vi "Teleop.vi"(10 "Match Info":T1={"Autonomous Elapsed Seconds"=0.0, "TeleOp Elapsed Seconds"=0.0, "Disabled Elapsed Seconds"=0.0, "Visited Autonomous"=FALSE, "Visited TeleOp"=FALSE, "Visited Disabled"=FALSE, "Autonomous Settings"={"Autonomous Style"=enum."Independent", "VI Refnum"=refnum}}, 11 "Call Context":T2) -> ()   [LabVIEW 2015]
doc: "This VI is called for each TeleOp packet received from the DS where the robot is not disabled. It is often used to read from the joysticks and update I/O or to update setpoints for timed control loops. It should complete and return within 20 milliseconds or it may miss DS packets."
uses:
  <vilib>/Rock Robotics/WPI/DriverStation/WPI_DriverStationDerivedRobotMode.ctl
  <vilib>/Rock Robotics/WPI/DriverStation/WPI_DriverStationMatch Info.ctl
  <vilib>/Rock Robotics/WPI/Solenoid/WPI_SolenoidValue.ctl
  <vilib>/Rock Robotics/WPI/Utilities/WPI_GetSetVariantRefNum.vi
  <vilib>/Rock Robotics/Network Tables/NT Write Boolean Array.vi
  <vilib>/Rock Robotics/Network Tables/NT Write Numeric Array.vi
  <vilib>/Rock Robotics/Network Tables/NT Read Boolean.vi
  <vilib>/Rock Robotics/Network Tables/NT Read Number.vi
  Robot Global Data.vi
  <vilib>/Rock Robotics/WPI/Solenoid/WPI_SolenoidSetEnum.vi
panel:
  out "Sample Slider 0":dbl(slide) scale=0.0..5.0
  out "Sample Boolean 1":bool
  out "Sample Boolean 0":bool
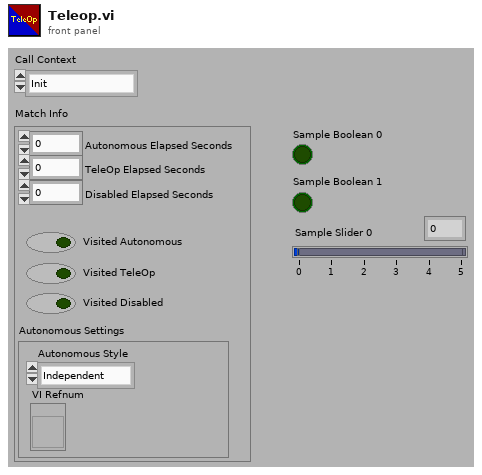
[diagram p1: front panel]
types:
  T1 = typedef "WPI_DriverStationMatch Info.ctl" = cluster{"Autonomous Elapsed Seconds":dbl, "TeleOp Elapsed Seconds":dbl, "Disabled Elapsed Seconds":dbl, "Visited Autonomous":bool, "Visited TeleOp":bool, "Visited Disabled":bool, "Autonomous Settings":cluster{"Autonomous Style":enum16{"Iterative", "Independent"}, "VI Refnum":refnum<vi>}}
  T2 = typedef "WPI_DriverStationDerivedRobotMode.ctl" = enum16{"Init", "Execute", "Stop"}
  T3 = typedef "WPI_JoystickDevRef.ctl" = cluster{"Device":T4}
  T4 = typedef "WPI_JoystickDeviceEnum.ctl" = enum16{"USB 0", "USB 1", "USB 2", "USB 3", "USB 4", "USB 5"}
  T5 = cluster{"Buttons[0]":bool, "Buttons[1]":bool, "Buttons[2]":bool, "Buttons[3]":bool, "Buttons[4]":bool, "Buttons[5]":bool, "Buttons[6]":bool, "Buttons[7]":bool, "Buttons[8]":bool}
  T6 = cluster{"Axes[0]":dbl, "Axes[1]":dbl, "Axes[2]":dbl, "Axes[3]":dbl, "Axes[4]":dbl, "Axes[5]":dbl, "Axes[6]":dbl, "Axes[7]":dbl, "Axes[8]":dbl}
  T7 = typedef "WPI_RobotDriveDevRef.ctl" = cluster{"DevStatus":errorcluster, "Motors[]":T8[], "Square Inputs":bool, "Max Output":dbl}
  T8 = typedef "WPI_MotorControlDeviceRef.ctl" = cluster{"DeviceStatus":errorcluster, "Type":T9, "PWM":cluster{"PWM Channel":T10, "DeadBand":T11}, "CAN":cluster{"Device Number":u8, "Control Mode":T12, "Semaphore":T13, "Max Vout":dbl, "TalonSRX Control Mode":T14}, "Invert":bool}
  T9 = typedef "WPI_MotorControlType.ctl" = enum16{"PWM", "CAN", "CANTalonSRX"}
  T10 = typedef "FPGA_DIOPWMChannel.ctl" = enum8{"PWM 0", "PWM 1", "PWM 2", "PWM 3", "PWM 4", "PWM 5", "PWM 6", "PWM 7", "PWM 8", "PWM 9", "PWM MXP 0", "PWM MXP 1", "PWM MXP 2", "PWM MXP 3", "PWM MXP 4", "PWM MXP 5", "PWM MXP 6", "PWM MXP 7", "PWM MXP 8", "PWM MXP 9", "Invalid"}
  T11 = typedef "WPI_PWMDeadband.ctl" = cluster{"Name":string, "maxPositivePwm":i32, "minPositivePwm":i32, "centerPwm":i32, "maxNegativePwm":i32, "minNegativePwm":i32, "angularRange":u16}
  T12 = typedef "WPI_CANJaguar_ControlMode.ctl" = enum8{"Percent VBus", "Current", "Speed", "Position", "Voltage"}
  T13 = typedef "Semaphore RefNum" = refnum<k1>
  T14 = typedef "WPI_CANTalonSRX_APIControlMode.ctl" = enum8{"Percent VBus", "Speed", "Position", "Slave", "Unchanged / Invalid", "Voltage Compensation", "Current", "Motion Profile"}
  T15 = typedef "WPI_SolenoidValue.ctl" = enum16{"Off", "On", "Forward", "Reverse"}
  T16 = typedef "WPI_SolenoidDevRef.ctl" = cluster{"DevStatus":errorcluster, "Pneumatics Control Module":u8, "Forward Solenoid Channel":T17, "Reverse Solenoid Channel":T17}
  T17 = typedef "WPI_SolenoidChannel.ctl" = enum8{"Solenoid 0", "Solenoid 1", "Solenoid 2", "Solenoid 3", "Solenoid 4", "Solenoid 5", "Solenoid 6", "Solenoid 7", "Invalid"}
  T18 = typedef "WPI_PotentiometerDevRef.ctl" = cluster{"DevStatus":errorcluster, "Analog Channel":T19, "Invert Output":bool}
  T19 = typedef "FPGA_AIChannel.ctl" = enum8{"AI 0", "AI 1", "AI 2", "AI 3", "AI MXP 0", "AI MXP 1", "AI MXP 2", "AI MXP 3", "Invalid"}
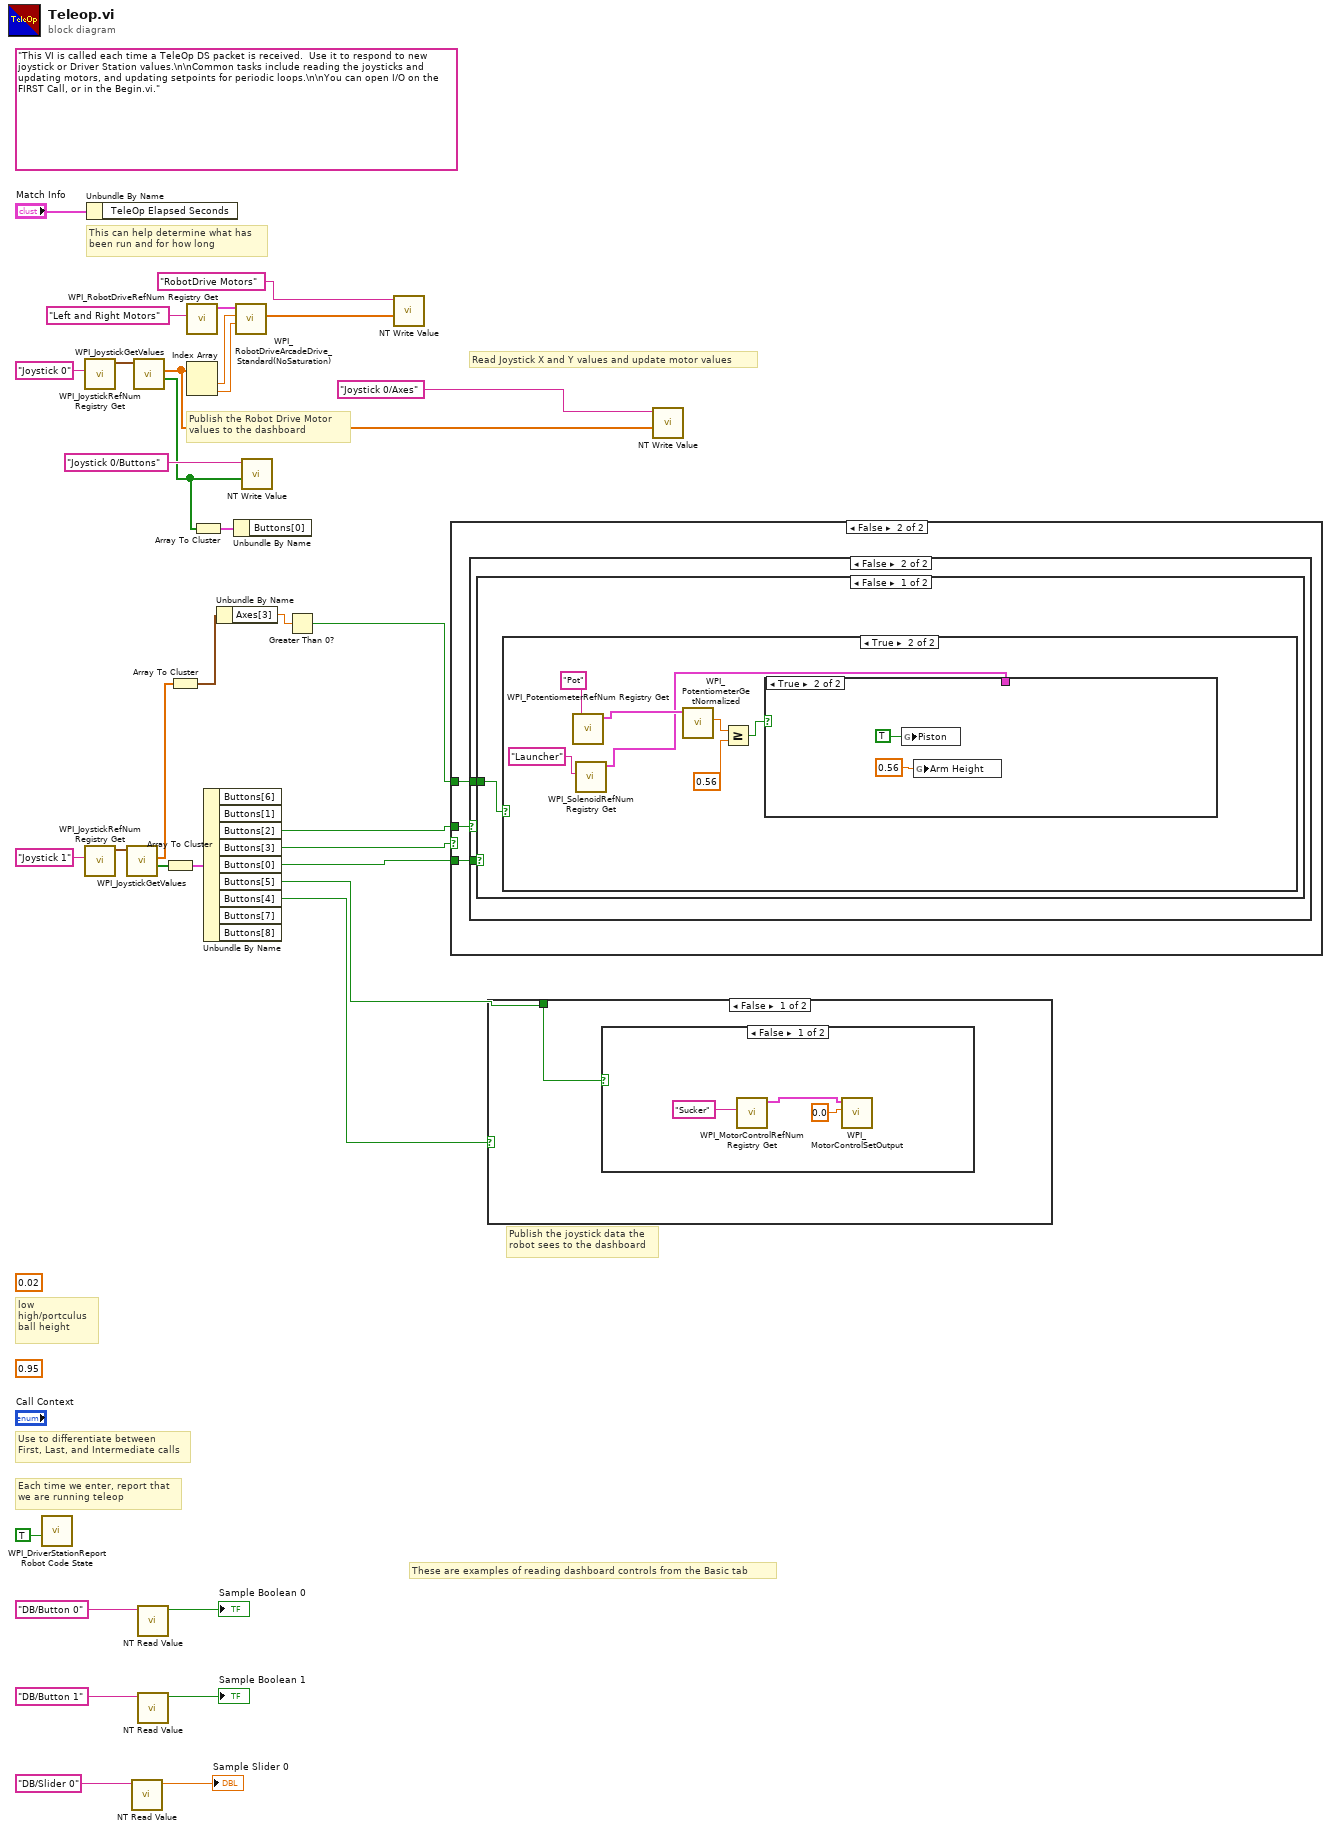
[diagram p0: block diagram]
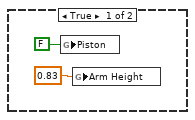
[diagram p2: hidden frame]
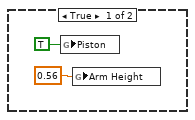
[diagram p3: hidden frame]
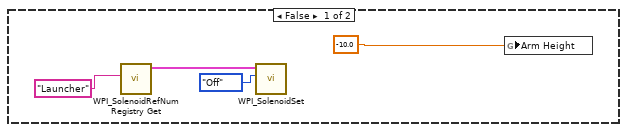
[diagram p4: hidden frame]
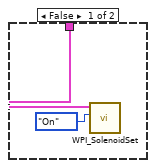
[diagram p5: hidden frame]
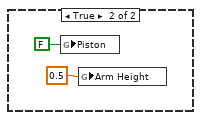
[diagram p6: hidden frame]
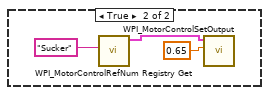
[diagram p7: hidden frame]
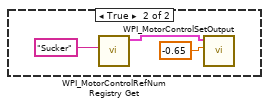
[diagram p8: hidden frame]
diagram:
  (unwired) 0.95 ("angle voltage")
  (unwired) 0.02 ("angle voltage")
  (unwired) "This VI is called each time a TeleOp DS packet is received.  Use it to respond to new joystick or Driver Station values.\n\nCommon tasks include reading the joysticks and updating motors, and updating setpoints for periodic loops.\n\nYou can open I/O on the FIRST Call, or in the Begin.vi."
  # "low\nhigh/portculus\nball height"
  # "These are examples of reading dashboard controls from the Basic tab"
  # "Publish the Robot Drive Motor\nvalues to the dashboard"
  # "Publish the joystick data the\nrobot sees to the dashboard"
  # "Each time we enter, report that\nwe are running teleop"
  # "Use to differentiate between\nFirst, Last, and Intermediate calls"
  # "This can help determine what has\nbeen run and for how long"
  # "Read Joystick X and Y values and update motor values"
  n1 = call <vilib>:"WPI_DriverStationReport Robot Code State.vi"("TeleOp"=TRUE ("Autonomous")) -> ()  [unwired: 10 in, 1 out]
  n2 = call <vilib>:"WPI_JoystickRefNum Registry Get.vi"("refnum name"="Joystick 0") -> ("JoystickDevRef"=w29:T3)  [unwired: 1 in, 9 out]
  n3 = call <vilib>:"WPI_JoystickRefNum Registry Get.vi"("refnum name"="Joystick 1") -> ("JoystickDevRef"=w13:T3)  [unwired: 9 in, 1 out]
  n4 = Unbundle By Name("Match Info") -> ()  [unwired: 1 out]
  n5 = call <vilib>:"WPI_JoystickGetValues.vi"("JoystickDevRef"=w13) -> ("Buttons"=w12:bool[], "Axes"=w3:dbl[])  [unwired: 6 in, 3 out]
  n6 = call-poly <vilib>:"NT Read Value.vi"("Name"="DB/Slider 0" ("refnum name")) -> ("Numeric"=→"Sample Slider 0":dbl)  [unwired: 9 in, 1 out]
  n7 = call <vilib>:"WPI_JoystickGetValues.vi"("JoystickDevRef"=w29) -> ("Buttons"=w9:bool[], "Axes"=w24:dbl[])  [unwired: 6 in, 3 out]
  n8 = call-poly <vilib>:"NT Read Value.vi"("Name"="DB/Button 0" ("refnum name")) -> ("Boolean"=→"Sample Boolean 0":bool)  [unwired: 9 in, 1 out]
  n9 = call-poly <vilib>:"NT Read Value.vi"("Name"="DB/Button 1" ("refnum name")) -> ("Boolean"=→"Sample Boolean 1":bool)  [unwired: 9 in, 1 out]
  n10 = Array To Cluster(array=w12) -> (cluster=w15:T5)
  n11 = Array To Cluster(array=w3) -> (cluster=w4:T6)
  n12 = call <vilib>:"WPI_RobotDriveRefNum Registry Get.vi"("refnum name"="Left and Right Motors") -> ("RobotDriveDevRef"=w32:T7)  [unwired: 1 in, 9 out]
  n13 = Index Array(array=w24) -> (element #1=w31:dbl, element #2=w27:dbl)  [unwired: 2 in]
  n14 = Array To Cluster(array=w9) -> (cluster=w8:T5)
  n15 = Unbundle By Name(w15) -> ("Buttons[2]"=w6:bool, "Buttons[3]"=w5:bool, "Buttons[0]"=w7:bool, "Buttons[5]"=w10:bool, "Buttons[4]"=w11:bool)  [unwired: 4 out]
  n16 = Unbundle By Name(w4) -> ("Axes[3]"=w2:dbl)
  n17 = Unbundle By Name(w8) -> ()  [unwired: 1 out]
  n18 = call <vilib>:"WPI_RobotDriveArcadeDrive_Standard(NoSaturation).vi"("Y axis value"=w27, "X axis value"=w31, "RobotDriveDevRef"=w32) -> ("Motor Values"=w17:dbl[])  [unwired: 1 in, 7 out]
  n19 = call-poly <vilib>:"NT Write Value.vi"("Boolean Array"=w9, "Name"="Joystick 0/Buttons") -> ()  [unwired: 9 in, 1 out]
  n20 = Greater Than 0?(x=w2) -> (x > 0?=w1:bool)
  n21 = call-poly <vilib>:"NT Write Value.vi"("Numeric Array"=w17, "Name"="RobotDrive Motors") -> ()  [unwired: 9 in, 1 out]
  n22 = case shown="False" w5 {
    tunnel: w6 -> [_ w39]
    tunnel: w7 -> [_ w38]
    tunnel: w1 -> [_ w37]
    frame True {
      n23 = global write "Robot Global Data.vi" "Piston"(FALSE) -> ()
      n24 = global write "Robot Global Data.vi" "Arm Height"(0.83 ("Arm Height")) -> ()
    }
    frame False {
      n25 = case shown="False" w39 {
        tunnel: w38 -> [_ w43]
        tunnel: w37 -> [_ w42]
        frame True {
          n26 = global write "Robot Global Data.vi" "Piston"(TRUE) -> ()
          n27 = global write "Robot Global Data.vi" "Arm Height"(0.56) -> ()
        }
        frame False {
          n28 = case shown="False" w43 {
            tunnel: w42 -> [w44 _]
            frame False {
              n29 = case shown="True" w44 {
                frame False {
                  n30 = call <vilib>:"WPI_SolenoidRefNum Registry Get.vi"("refnum name"="Launcher") -> ("SolenoidDevRef"=w48:T16)  [unwired: 9 in, 1 out]
                  n31 = call-poly <vilib>:"WPI_SolenoidSet.vi"("Value"=WPI_SolenoidValue."Off", "SolenoidDevRef"=w48) -> ()  [unwired: 8 in, 2 out]
                  n32 = global write "Robot Global Data.vi" "Arm Height"(-10.0) -> ()
                }
                frame True {
                  n33 = call <vilib>:"WPI_PotentiometerRefNum Registry Get.vi"("refnum name"="Pot") -> ("PotDevRef"=w50:T18)  [unwired: 9 in, 1 out]
                  n34 = call <vilib>:"WPI_SolenoidRefNum Registry Get.vi"("refnum name"="Launcher") -> ("SolenoidDevRef"=w49:T16)  [unwired: 9 in, 1 out]
                  n35 = call <vilib>:"WPI_PotentiometerGetNormalized.vi"("PotDevRef"=w50) -> ("Normalized Value"=w53:dbl)  [unwired: 8 in, 2 out]
                  n36 = Greater Or Equal?(x=w53, y=0.56) -> (x >= y?=w51:bool)
                  n37 = case shown="True" w51 {
                    tunnel: w49 -> [w56 _]
                    frame False {
                      n38 = call-poly <vilib>:"WPI_SolenoidSet.vi"("Value"=WPI_SolenoidValue."On", "SolenoidDevRef"=w56) -> ()  [unwired: 8 in, 2 out]
                    }
                    frame True {
                      n39 = global write "Robot Global Data.vi" "Piston"(TRUE) -> ()
                      n40 = global write "Robot Global Data.vi" "Arm Height"(0.56) -> ()
                    }
                  }
                }
              }
            }
            frame True {
              n41 = global write "Robot Global Data.vi" "Piston"(FALSE) -> ()
              n42 = global write "Robot Global Data.vi" "Arm Height"(0.5 ("Arm Height")) -> ()
            }
          }
        }
      }
    }
  }
  n43 = case shown="False" w11 {
    tunnel: w10 -> [w62 _]
    frame False {
      n44 = case shown="False" w62 {
        frame False {
          n45 = call <vilib>:"WPI_MotorControlRefNum Registry Get.vi"("refnum name"="Sucker") -> ("MotorControlDevRef"=w64:T8)  [unwired: 9 in, 1 out]
          n46 = call <vilib>:"WPI_MotorControlSetOutput.vi"("Output"=0.0, "MotorControlDevRef"=w64) -> ()  [unwired: 7 in, 3 out]
        }
        frame True {
          n47 = call <vilib>:"WPI_MotorControlRefNum Registry Get.vi"("refnum name"="Sucker") -> ("MotorControlDevRef"=w67:T8)  [unwired: 9 in, 1 out]
          n48 = call <vilib>:"WPI_MotorControlSetOutput.vi"("Output"=0.65, "MotorControlDevRef"=w67) -> ()  [unwired: 7 in, 3 out]
        }
      }
    }
    frame True {
      n49 = call <vilib>:"WPI_MotorControlRefNum Registry Get.vi"("refnum name"="Sucker") -> ("MotorControlDevRef"=w70:T8)  [unwired: 9 in, 1 out]
      n50 = call <vilib>:"WPI_MotorControlSetOutput.vi"("Output"=-0.65, "MotorControlDevRef"=w70) -> ()  [unwired: 7 in, 3 out]
    }
  }
  n51 = call-poly <vilib>:"NT Write Value.vi"("Numeric Array"=w24, "Name"="Joystick 0/Axes") -> ()  [unwired: 9 in, 1 out]
